vi "Read IO State.vi"(8 "error in":errorcluster, 11 "PLC in":refnum<class "PLC.lvclass">) -> (0 "error out":errorcluster, 3 "PLC out":refnum<class "PLC.lvclass">)   [LabVIEW 2018, in "PLC.lvlib" / "PLC.lvclass"]
uses:
  PLC.lvclass
  Custom Controls/Selector.ctl
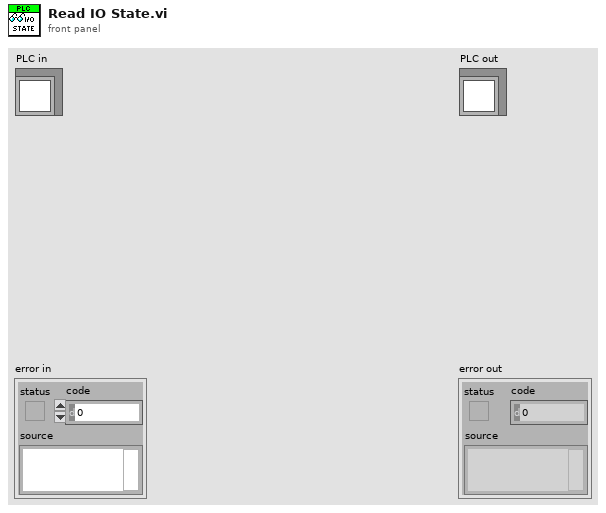
[diagram p1: front panel]
types:
  T1 = typedef "PLC.lvlib/PLC.lvclass/Selector.ctl" = enum16{"Digital", "Analog"}
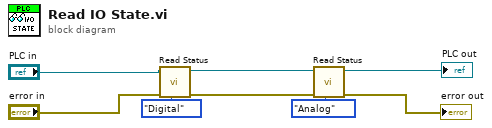
[diagram p0: block diagram]
diagram:
  n1 = call-dynamic "Read Status.vi"("Selector"=Selector."Digital", "error in"="error in", "PLC in"="PLC in") -> ("error out"=w4:errorcluster, "PLC out"=w5:refnum<class "PLC.lvclass">)  [unwired: 7 in]
  n2 = call-dynamic "Read Status.vi"("Selector"=Selector."Analog", "error in"=w4, "PLC in"=w5) -> ("error out"=→"error out":errorcluster, "PLC out"=→"PLC out":refnum<class "PLC.lvclass">)  [unwired: 7 in]
